vi "Export Resources to File.vi"(8 "error in (no error)":errorcluster, 10 "File Path":path, 11 "LangFile.lvclass in":refnum<class "Resource Data.lvclass">) -> (0 "error out":errorcluster, 3 "LangFile.lvclass out":refnum<class "Resource Data.lvclass">)   [LabVIEW 2013, in "SET Project Data.lvlib" / "Resource Data.lvclass"]
uses:
  Resource Data.lvclass
  Resource Data.lvclass/Resource Data.ctl
  Read Resources.vi
  Read Languages.vi
  Lib/Robust CSV/Write CSV File_1D (UTF-16).vi
  Lib/Robust CSV/Write CSV File_2D (UTF-16).vi
  Lib/Robust CSV/SET_Robust CSV (UTF-16).lvlib
  Lib/Unicode/SET_Unicode Tools.lvlib
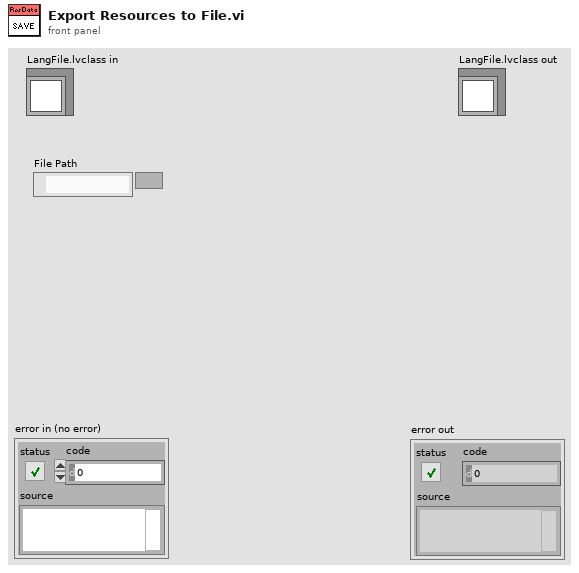
[diagram p1: front panel]
types:
  T1 = typedef "SET Project Data.lvlib/ProjFile_Resource Data.ctl" = cluster{"RID":string, "Tag":string, "Strings [] (UTF-16)":string[], "Shared?":bool}
  T2 = typedef "SET Project Data.lvlib/ProjFile_Language Data.ctl" = cluster{"Tag":string, "Name":string, "Code Page":u16}
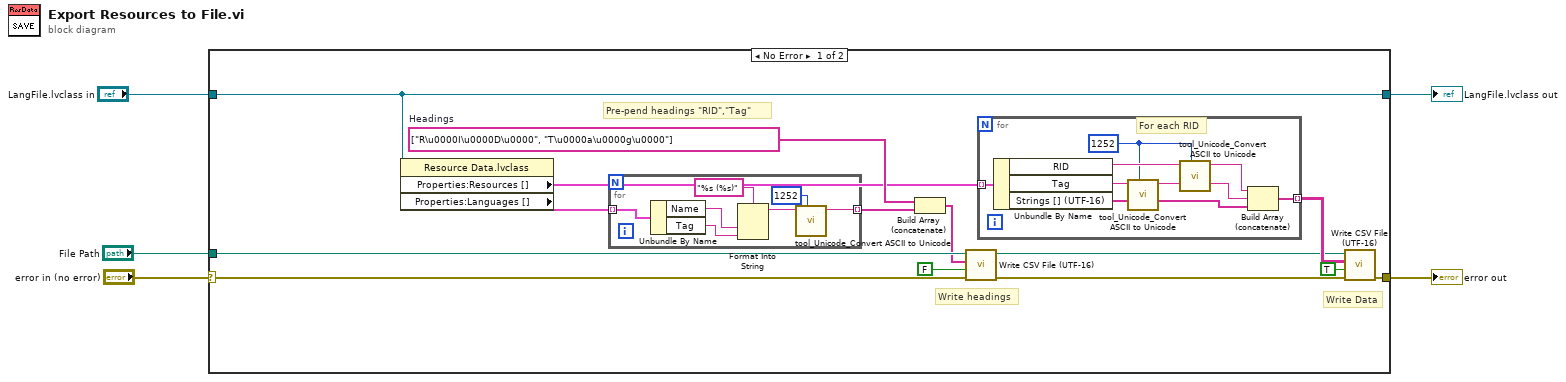
[diagram p0: block diagram]
diagram:
  n1 = case shown="No Error" "error in (no error)" {
    selector: "error in (no error)" -> [w16 w36]
    tunnel: [w9 w36] -> w5
    tunnel: "File Path" -> [w17 _]
    tunnel: "LangFile.lvclass in" -> [w6 w35]
    tunnel: [w6 w35] -> w4
    frame No Error {
      w19 = string[] ["R\u0000I\u0000D\u0000", "T\u0000a\u0000g\u0000"]  # Headings
      # "Write Data"
      # "Write headings"
      # "Pre-pend headings \"RID\",\"Tag\""
      n2 = property class="Resource Data.lvclass"(reference=w6) -> ("Properties:Resources []"=w8:T1[], "Properties:Languages []"=w7:T2[])  [unwired: 1 in, 2 out]
      n3 = for {
        tunnel: w7 -> [w26] mode=indexing
        tunnel: [w21] -> w18 mode=indexing
        n4 = Unbundle By Name(w26) -> ("Name"=w24:string, "Tag"=w23:string)
        n5 = Format Into String(format string="%s (%s)", w24, w23) -> (resulting string=w22:string)  [unwired: 2 in, 1 out]
        n6 = call "tool_Unicode_Convert ASCII to Unicode.vi"("Source Code Page"=u16 1252, "MultiByteStr (ANSI)"=w22) -> ("WideCharStr (UTF-16LE)"=w21:string)  [unwired: 8 in, 1 out]
      }
      n7 = Build Array (concatenate)(w19, w18) -> (w15:string[])
      n8 = call-poly "Write CSV File (UTF-16).vi"("error in (no error)"=w16, "append to file? (new file)"=FALSE, "1D array *UTF-16"=w15, "file path in"=w17) -> ("error out"=w12:errorcluster, "file path out"=w10:path)  [unwired: 6 in]
      n9 = for {
        tunnel: w8 -> [w34] mode=indexing
        tunnel: [w32] -> w13 mode=indexing
        w27 = u16 1252 ("Source Code Page")
        # "For each RID"
        n10 = Unbundle By Name(w34) -> ("RID"=w31:string, "Tag"=w29:string, "Strings [] (UTF-16)"=w33:string[])
        n11 = call "tool_Unicode_Convert ASCII to Unicode.vi"("Source Code Page"=w27, "MultiByteStr (ANSI)"=w29) -> ("WideCharStr (UTF-16LE)"=w28:string)  [unwired: 8 in, 1 out]
        n12 = call "tool_Unicode_Convert ASCII to Unicode.vi"("Source Code Page"=w27, "MultiByteStr (ANSI)"=w31) -> ("WideCharStr (UTF-16LE)"=w30:string)  [unwired: 8 in, 1 out]
        n13 = Build Array (concatenate)(w30, w28, w33) -> (w32:string[])
      }
      n14 = call-poly "Write CSV File (UTF-16).vi"("error in (no error)"=w12, "append to file? (new file)"=TRUE, "2D array *UTF-16"=w13, "file path in"=w10) -> ("error out"=w9:errorcluster)  [unwired: 6 in, 1 out]
    }
    frame Error {
    }
  }
  "error out" <- w5
  "LangFile.lvclass out" <- w4
